vi "Column Type.vi"(8 "error in (no error)":errorcluster, 11 "SQL Statement in":refnum<class "SQL Statement.lvclass">) -> (0 "error out":errorcluster, 2 "SQLite3 type":T1, 3 "SQL Statement out":refnum<class "SQL Statement.lvclass">)   [LabVIEW 2013, in "SQLiteSupport.lvlib" / "SQL Statement.lvclass"]
doc: "Gets the SQLite3 datatype of the value stored in the column. Not that different entries in a column can have diffferent types."
uses:
  SQL Statement.lvclass
  SQLITE Datatype.ctl
  SQL Statement.lvclass/SQL Statement.ctl
  SQLiteSupport.lvlib
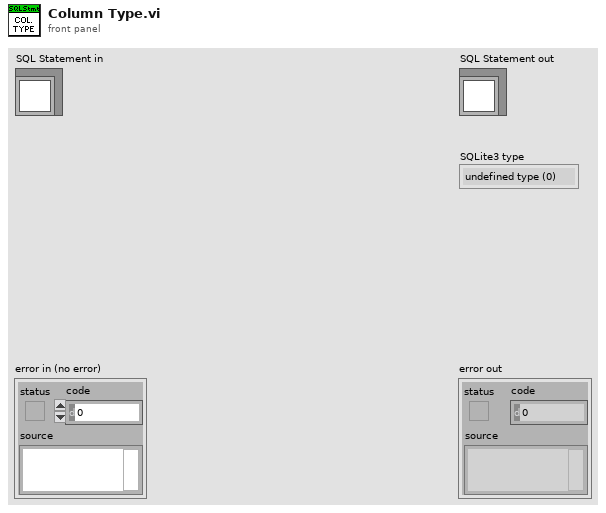
[diagram p1: front panel]
types:
  T1 = typedef "SQLiteSupport.lvlib/SQLITE Datatype.ctl" = enum32{"undefined type (0)", "SQLITE_INTEGER", "SQLITE_FLOAT", "SQLITE3_TEXT", "SQLITE_BLOB", "SQLITE_NULL", "undefined type"}
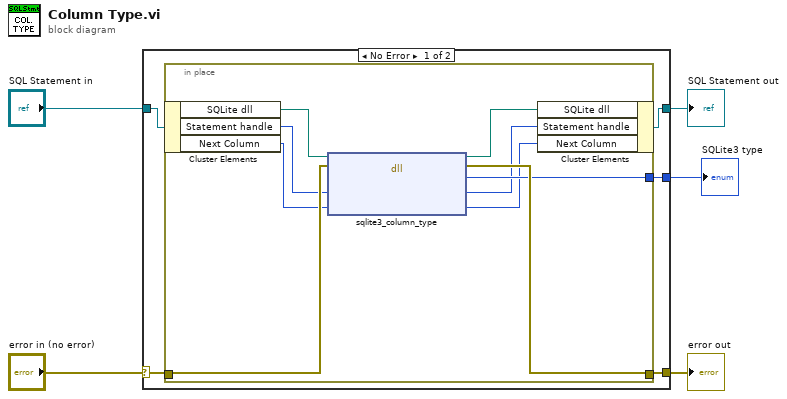
[diagram p0: block diagram]
diagram:
  n1 = case shown="No Error" "error in (no error)" {
    selector: "error in (no error)" -> [w10 w21]
    tunnel: [w9 w21] -> w4
    tunnel: [w6 w20] -> w2
    tunnel: "SQL Statement in" -> [w7 w20]
    tunnel: [w8 _] -> w1
    frame No Error {
      n2 = in-place {
        in-place-border: w10 -> [w19]
        in-place-border: [w18] -> w9
        in-place-border: [w17] -> w8
        n3 = in-place-cluster #1(w7) -> ("SQLite dll"=w14:path, "Statement handle"=w15:u64, "Next Column"=w16:i32)
        n4 = dll-call lib="C:/LabVIEW_JDP/Support/SQLite/sqlite3.dll" fn="sqlite3_column_type"(path in=w14, error in=w19, "Statement"=w15, "Column"=w16) -> (path out=w13:path, error out=w18:errorcluster, "Type"=w17:u32, "Statement"=w12:u64, "Column"=w11:i32)  [unwired: 1 in]
        n5 = in-place-cluster #1("SQLite dll"=w13, "Statement handle"=w12, "Next Column"=w11) -> (w6:refnum<class "SQL Statement.lvclass">)
      }
    }
    frame Error {
    }
  }
  "error out" <- w4
  "SQL Statement out" <- w2
  "SQLite3 type" <- w1
